vi "DriveReadEncoder.vi"(8 "error in":errorcluster, 11 "ModualNamePrefix":i32) -> (0 "error out":errorcluster, 2 "SWERVE_DRIVE_MODULE_POSITION":T1={"Distance"=0.0, "Angle"={"VALUE"=0.0, "COS"=1.0, "SIN"=0.0}, "P"=FALSE} {"Angle"."SIN" format="%13.4f"; "Angle"."COS" format="%13.4f"; "Angle"."VALUE" format="%13.4f"}, 3 "SWERVE_DRIVE_MODULE_STATE":T3={"Speed"=0.0, "Angle"={"VALUE"=0.0, "COS"=1.0, "SIN"=0.0}} {"Angle"."SIN" format="%13.4f"; "Angle"."COS" format="%13.4f"; "Angle"."VALUE" format="%13.4f"})   [LabVIEW 2023]
uses:
  <vilib>/Rock Robotics/WPI/ThirdParty/JAS_Junk/TrajLib/TypeDef/SWERVE_DRIVE_MODULE_STATE.ctl
  <vilib>/Rock Robotics/WPI/ThirdParty/JAS_Junk/TrajLib/TypeDef/ROTATION2D.ctl
  <vilib>/Rock Robotics/WPI/ThirdParty/JAS_Junk/TrajLib/TypeDef/SWERVE_DRIVE_MODULE_POSITION.ctl
  <vilib>/Rock Robotics/WPI/ThirdParty/JAS_Junk/TrajLib/Conv_Deg_Radians.vi
  <vilib>/Rock Robotics/WPI/ThirdParty/JAS_Junk/TrajLib/Rotation2d_CreateAngle.vi
  <vilib>/Rock Robotics/WPI/ThirdParty/JAS_Junk/TrajLib/LinearFilter_ResetToValue.vi
  <vilib>/Rock Robotics/WPI/ThirdParty/JAS_Junk/TrajLib/LinearFilter_Calculate.vi
  DriveGlobal.vi
  <vilib>/Rock Robotics/WPI/ThirdParty/Phoenix-LabVIEW/CANCoder/CTRE_Phoenix_CANcoder_RefNumRegistryGet.vi
  <vilib>/Rock Robotics/WPI/MotorControl/WPI_MotorControlRefNum Registry Get.vi
  <vilib>/Rock Robotics/WPI/ThirdParty/JAS_Junk/TrajLib/LinearFilter_MovingAverage.vi
  <vilib>/Rock Robotics/WPI/ThirdParty/JAS_Junk/TrajLib/LinearFilter_LowPassBW1.vi
  <vilib>/Rock Robotics/WPI/ThirdParty/JAS_Junk/TrajLib/LinearFilter_LowPassBW2.vi
  <vilib>/Rock Robotics/WPI/ThirdParty/JAS_Junk/TrajLib/LinearFilter_HighPassBW1.vi
  <vilib>/Rock Robotics/WPI/ThirdParty/JAS_Junk/TrajLib/LinearFilter_HighPassBW2.vi
  <vilib>/Rock Robotics/WPI/ThirdParty/Phoenix-LabVIEW/CANCoder/Get/CTRE_Phoenix_CANcoder_GetSensorData.vi
  <vilib>/Rock Robotics/Network Tables/NT Write Number.vi
  <vilib>/Rock Robotics/WPI/ThirdParty/JAS_Junk/TrajLib/Trajectory_Library.lvlib
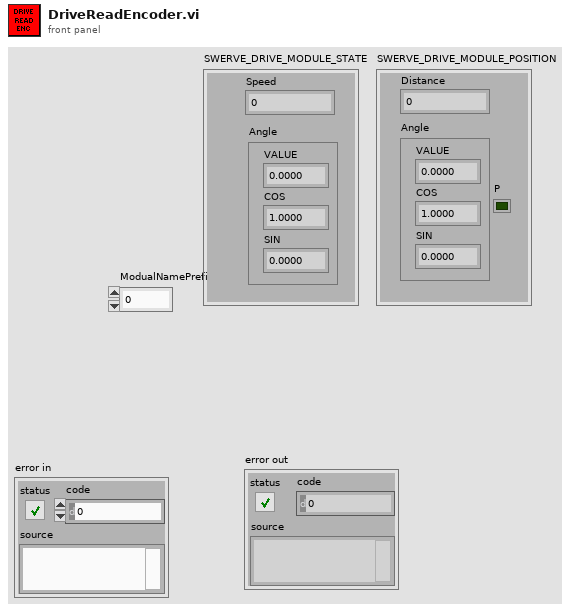
[diagram p1: front panel]
types:
  T1 = typedef "Trajectory_Library.lvlib/SWERVE_DRIVE_MODULE_POSITION.ctl" = cluster{"Distance":dbl, "Angle":T2, "P":bool}
  T2 = typedef "Trajectory_Library.lvlib/ROTATION2D.ctl" = cluster{"VALUE":dbl, "COS":dbl, "SIN":dbl}
  T3 = typedef "Trajectory_Library.lvlib/SWERVE_DRIVE_MODULE_STATE.ctl" = cluster{"Speed":dbl, "Angle":T2}
  T4 = enum16{"Moving Average", "Low Pass 1st Order Butterworth", "Low Pass 2nd Order Butterworth", "High Pass 1st Order Butterworth", "High Pass 2nd Order Butterworth"}
  T5 = typedef "WPI_MotorControlDeviceRef.ctl" = cluster{"DeviceStatus":errorcluster, "Type":T6, "PWM":cluster{"PWM Channel":T7, "DeadBand":T8}, "CAN":cluster{"Device Number":u8, "SetOutput VI Ref":variant, "GetOutput VI Ref":variant, "Enable VI Ref":variant, "Disable VI Ref":variant, "Data":variant}, "Invert":bool, "DIO PWM":cluster{"PWM \"Enable\" Channel":T7, "DIOChannel":T9, "PWM Rate":dbl}}
  T6 = typedef "WPI_MotorControlType.ctl" = enum16{"PWM", "CAN", "DIO PWM"}
  T7 = typedef "FPGA_DIOPWMChannel.ctl" = enum8{"PWM 0", "PWM 1", "PWM 2", "PWM 3", "PWM 4", "PWM 5", "PWM 6", "PWM 7", "PWM 8", "PWM 9", "PWM MXP 0", "PWM MXP 1", "PWM MXP 2", "PWM MXP 3", "PWM MXP 4", "PWM MXP 5", "PWM MXP 6", "PWM MXP 7", "PWM MXP 8", "PWM MXP 9", "Invalid"}
  T8 = typedef "WPI_PWMDeadband.ctl" = cluster{"Name":string, "maxPositivePwm":i32, "minPositivePwm":i32, "centerPwm":i32, "maxNegativePwm":i32, "minNegativePwm":i32, "angularRange":u16}
  T9 = typedef "FPGA_DIOChannel.ctl" = enum8{"DIO 0", "DIO 1", "DIO 2", "DIO 3", "DIO 4", "DIO 5", "DIO 6", "DIO 7", "DIO 8", "DIO 9", "DIO MXP 0", "DIO MXP 1", "DIO MXP 2", "DIO MXP 3", "DIO MXP 4", "DIO MXP 5", "DIO MXP 6", "DIO MXP 7", "DIO MXP 8", "DIO MXP 9", "DIO MXP 10", "DIO MXP 11", "DIO MXP 12", "DIO MXP 13", "DIO MXP 14", "DIO MXP 15", "SPI Port CS1", "SPI Port CS2", "SPI Port CS3", "SPI Port MISO", "SPI Port MOSI", "Invalid"}
  T10 = typedef "CTRE_Phoenix_CANcoder_DeviceRef.ctl" = cluster{"DeviceStatus":errorcluster, "Device Number":u8, "Handle":u64, "UsageFrame":u32, "Library Path":path}
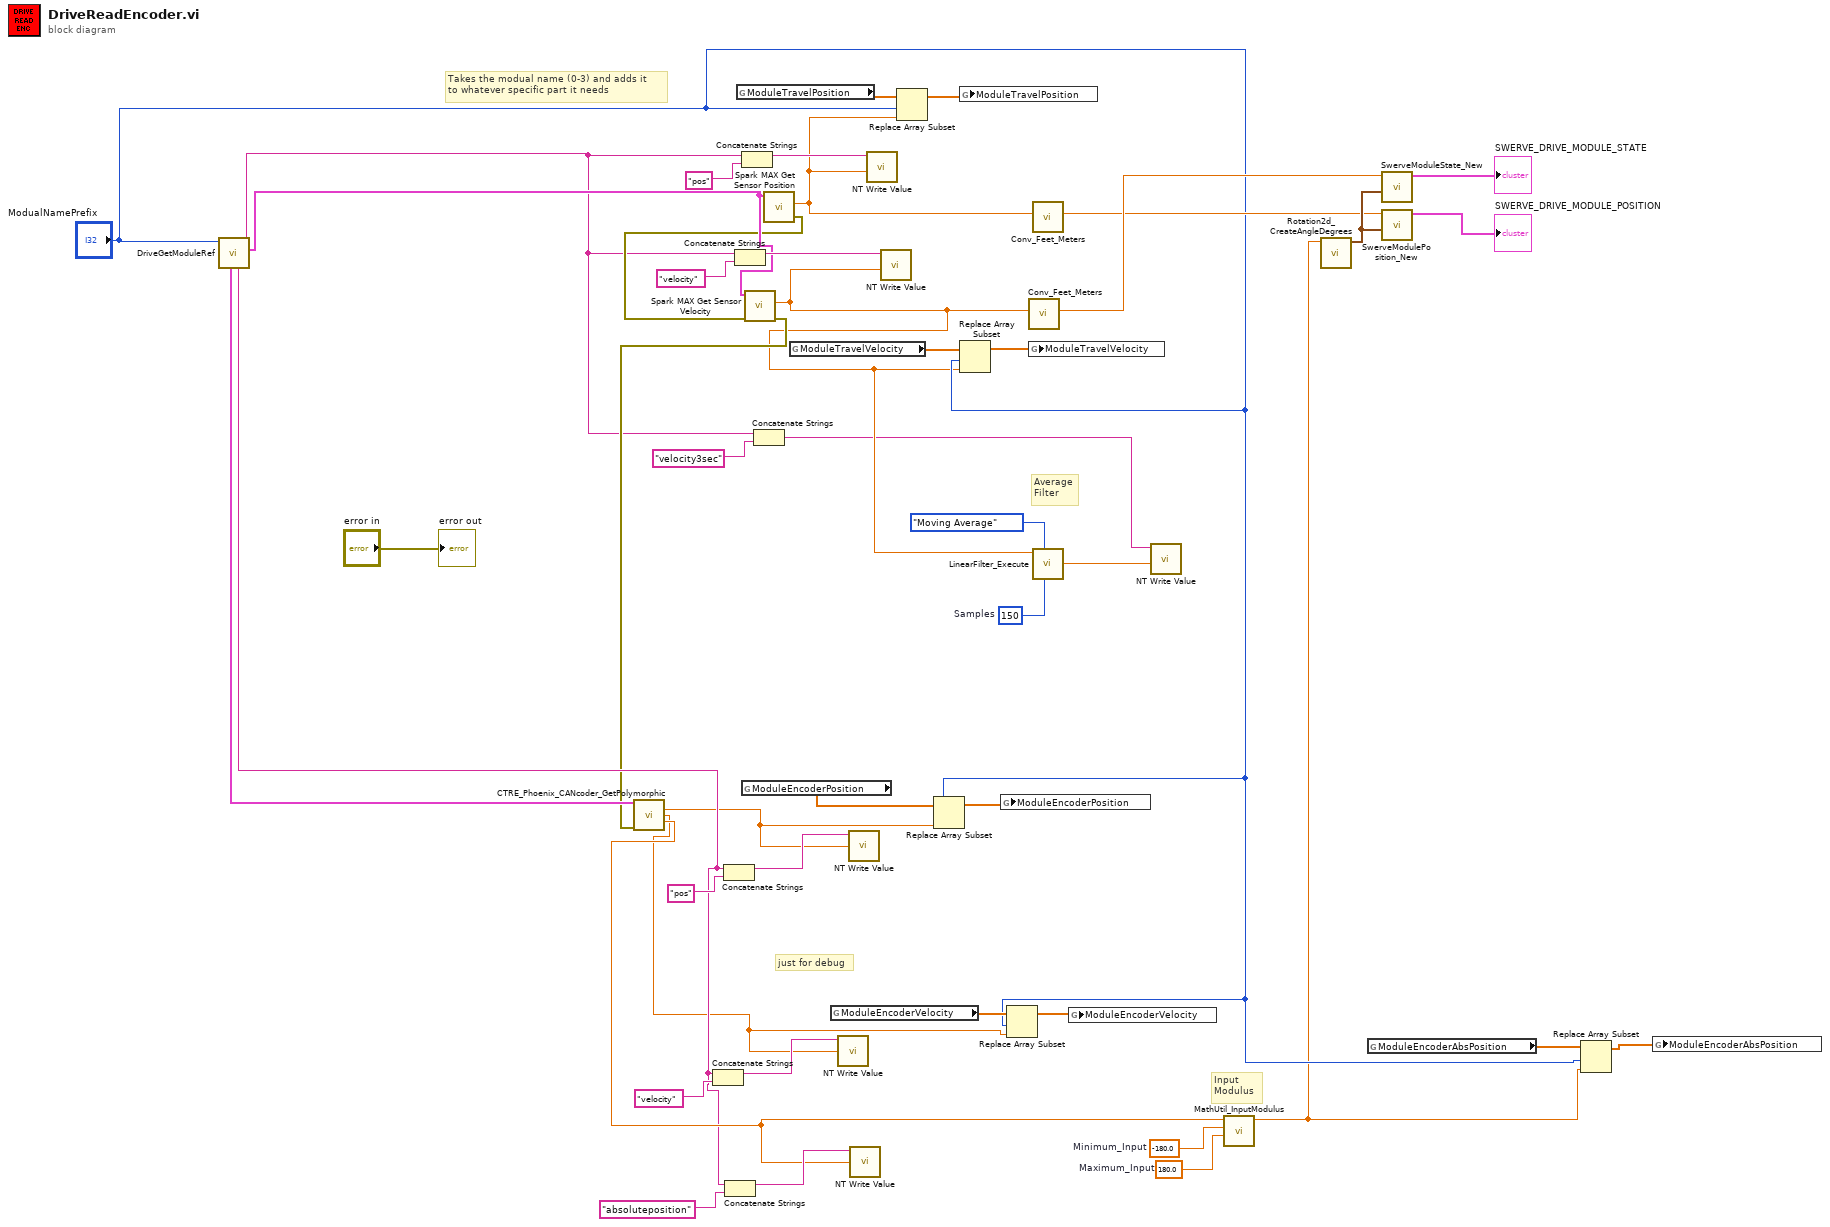
[diagram p0: block diagram]
diagram:
  w5 = 150  # Samples
  w31 = -180.0  # Minimum_Input
  w30 = 180.0  # Maximum_Input
  # "Average\nFilter"
  # "Input\nModulus"
  # "just for debug"
  # "Takes the modual name (0-3) and adds it \nto whatever specific part it needs"
  n1 = call "DriveGetModuleRef.vi"("ModualNamePrefix"="ModualNamePrefix") -> ("TravMot"=w35:T5, "TravStr"=w6:string, "EncStr"=w23:string, "EncDevice"=w22:T10)  [unwired: 5 in, 2 out]
  n2 = Concatenate Strings(w23, "velocity" ("refnum name")) -> (w42:string)
  n3 = Concatenate Strings(w23, "pos" ("refnum name")) -> (w44:string)
  n4 = Concatenate Strings(w23, "absoluteposition" ("refnum name")) -> (w40:string)
  n5 = Concatenate Strings(w6, "velocity" ("refnum name")) -> (w36:string)
  n6 = global read "DriveGlobal.vi" "ModuleTravelPosition"() -> (w26:dbl[])
  n7 = Concatenate Strings(w6, "pos" ("refnum name")) -> (w38:string)
  n8 = global read "DriveGlobal.vi" "ModuleEncoderPosition"() -> (w19:dbl[])
  n9 = Concatenate Strings(w6, "velocity3sec" ("refnum name")) -> (w2:string)
  n10 = call <vilib>:"Spark MAX Get Sensor Position.vi"("MotorControlDevRef in"=w35) -> ("error out"=w9:errorcluster, "Sensor Position"=w24:dbl)  [unwired: 7 in, 2 out]
  n11 = call <vilib>:"Spark MAX Get Sensor Velocity.vi"("error in (no error)"=w9, "MotorControlDevRef in"=w35) -> ("error out"=w8:errorcluster, "Sensor Velocity"=w3:dbl)  [unwired: 6 in, 2 out]
  n12 = call-poly <vilib>:"CTRE_Phoenix_CANcoder_GetPolymorphic.vi"("CTRE_CANcoder_DeviceRef"=w22, "error in"=w8) -> ("Position"=w17:dbl, "Velocity"=w14:dbl, "Absolute Position"=w29:dbl)  [unwired: 9 in, 2 out]
  n13 = global read "DriveGlobal.vi" "ModuleTravelVelocity"() -> (w21:dbl[])
  n14 = global read "DriveGlobal.vi" "ModuleEncoderVelocity"() -> (w16:dbl[])
  n15 = call-poly <vilib>:"NT Write Value.vi"("value"=w14, "name"=w42) -> ()  [unwired: 9 in, 1 out]
  n16 = call-poly <vilib>:"NT Write Value.vi"("value"=w17, "name"=w44) -> ()  [unwired: 9 in, 1 out]
  n17 = call-poly <vilib>:"NT Write Value.vi"("value"=w29, "name"=w40) -> ()  [unwired: 9 in, 1 out]
  n18 = call-poly <vilib>:"NT Write Value.vi"("value"=w24, "name"=w38) -> ()  [unwired: 9 in, 1 out]
  n19 = call-poly <vilib>:"NT Write Value.vi"("value"=w3, "name"=w36) -> ()  [unwired: 9 in, 1 out]
  n20 = Replace Array Subset(array=w26, new element=w24, index="ModualNamePrefix") -> (w25:dbl[])
  n21 = Replace Array Subset(array=w19, new element=w17, index="ModualNamePrefix") -> (w18:dbl[])
  n22 = global write "DriveGlobal.vi" "ModuleTravelPosition"(w25) -> ()
  n23 = Replace Array Subset(array=w21, new element=w3, index="ModualNamePrefix") -> (w20:dbl[])
  n24 = global write "DriveGlobal.vi" "ModuleEncoderPosition"(w18) -> ()
  n25 = Replace Array Subset(array=w16, new element=w14, index="ModualNamePrefix") -> (w15:dbl[])
  n26 = call <vilib>:"Conv_Feet_Meters.vi"("Feet"=w3) -> ("Meters"=w28:dbl)  [unwired: 10 in]
  n27 = global write "DriveGlobal.vi" "ModuleTravelVelocity"(w20) -> ()
  n28 = call <vilib>:"Conv_Feet_Meters.vi"("Feet"=w24) -> ("Meters"=w27:dbl)  [unwired: 10 in]
  n29 = call <vilib>:"LinearFilter_Execute.vi"("Samples"=w5, "Filter Type"=T4."Moving Average", "Input"=w3) -> ("Output"=w1:dbl)  [unwired: 7 in, 1 out]
  n30 = global write "DriveGlobal.vi" "ModuleEncoderVelocity"(w15) -> ()
  n31 = call-poly <vilib>:"NT Write Value.vi"("value"=w1, "name"=w2) -> ()  [unwired: 9 in, 1 out]
  n32 = call <vilib>:"MathUtil_InputModulus.vi"("Maximum_Input"=w30, "Minimum_Input"=w31, "Input"=w29) -> ("modulus"=w10:dbl)  [unwired: 8 in]
  n33 = call <vilib>:"Rotation2d_CreateAngleDegrees.vi"("Angle_Degrees"=w10) -> ("ROTATION"=w34:T2)  [unwired: 10 in]
  n34 = global read "DriveGlobal.vi" "ModuleEncoderAbsPosition"() -> (w13:dbl[])
  n35 = call <vilib>:"SwerveModuleState_New.vi"("ROTATION"=w34, "Speed"=w28) -> ("SWERVE_DRIVE_MODULE_STATE"=→"SWERVE_DRIVE_MODULE_STATE":T3)  [unwired: 9 in]
  n36 = call <vilib>:"SwerveModulePosition_New.vi"("ROTATION"=w34, "Distance"=w27) -> ("SWERVE_DRIVE_MODULE_POSITION"=→"SWERVE_DRIVE_MODULE_POSITION":T1)  [unwired: 9 in]
  n37 = Replace Array Subset(array=w13, new element=w10, index="ModualNamePrefix") -> (w12:dbl[])
  n38 = global write "DriveGlobal.vi" "ModuleEncoderAbsPosition"(w12) -> ()
  "error out" <- "error in"
